vi "Host-Top-Level.vi"() -> ()   [LabVIEW 2015]
uses:
  <vilib>/rvi/interface/RandomDataEmulation/nirviRandomDataOpen.vi
  <vilib>/rvi/interface/common/niFpgaCacheSessionInfoDynamic.vi
  <vilib>/Utility/error.llb/Error Cluster From Error Code.vi
  <vilib>/rvi/errors/niLvFpgaAdjustHostInterfaceError.vi
  <vilib>/FPGAPlugInAG/Dynamic/niLvFpga_Close_Dynamic.vi
  <vilib>/rvi/interface/nirviOpenFPGA/nirviOpenFPGA.xnode
  FPGA-SRAM-Top-Level.vi
  <vilib>/rvi/interface/nirviMethod/nirviMethod.xnode
  <vilib>/rvi/interface/nirviCloseFPGA/nirviCloseFPGA.xnode
  <vilib>/FPGAPlugInAG/Dynamic/niLvFpga_WriteFifo_Dynamic.vi
  <vilib>/rvi/errors/niLvFpgaMergeErrorWithErrorCode.vi
  <vilib>/FPGAPlugInAG/Dynamic/niLvFpga_ReadFifo_Dynamic.vi
panel:
  out "error out":errorcluster
  in  "error in":errorcluster
  in  "# of \nElements":u32=2
  in  "Start\nAddress":u32
  out "Data Out":u64[](array[numeric])
  in  "Write Memory":bool
  in  "Data":u64[](array[numeric])=[10, 11, 12, 13, 14]
  in  "Exit":bool
  in  "Read Memory":bool
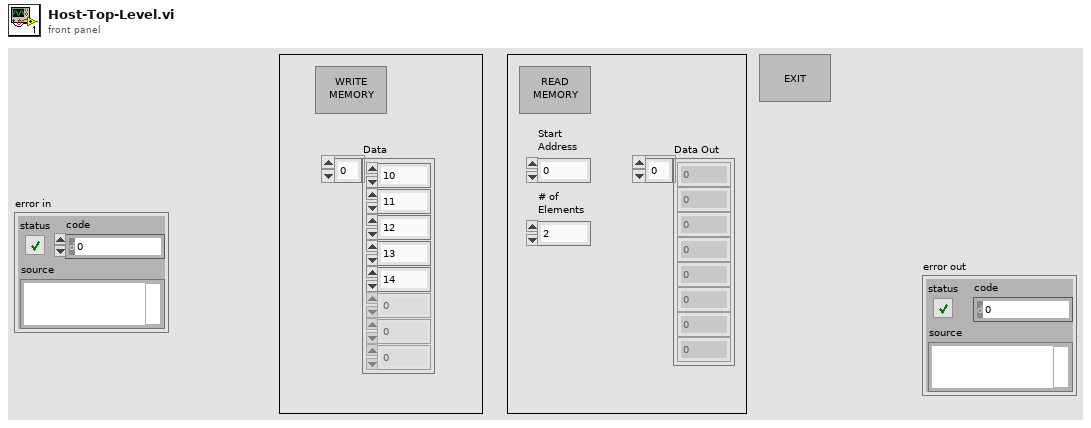
[diagram p1: front panel]
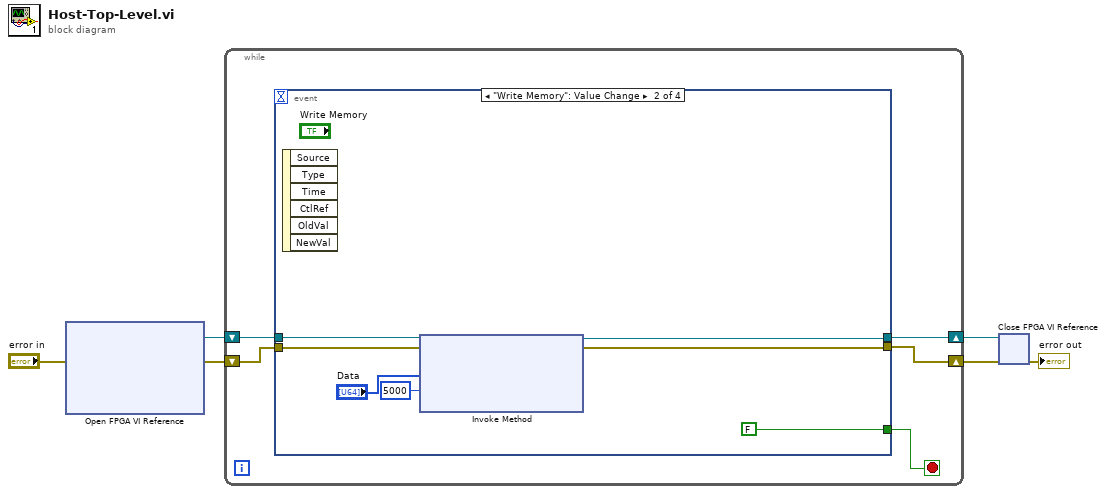
[diagram p0: block diagram]
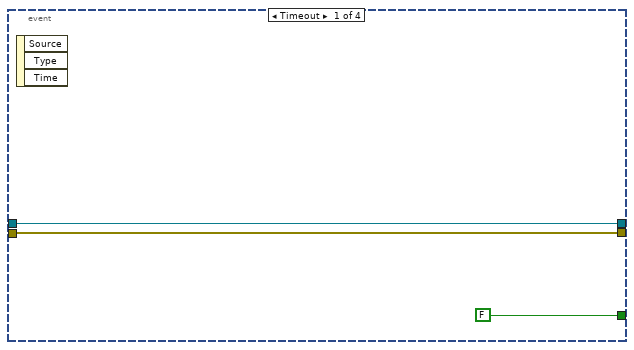
[diagram p2: hidden frame]
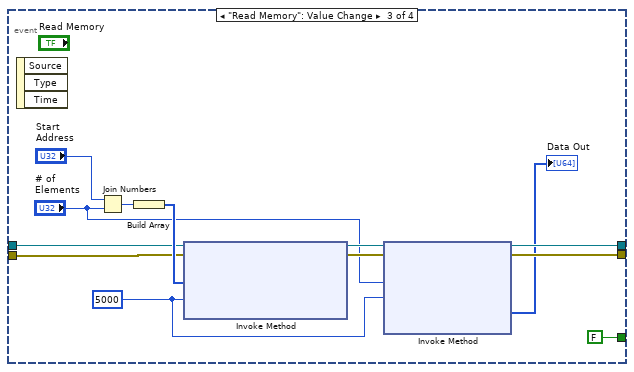
[diagram p3: hidden frame]
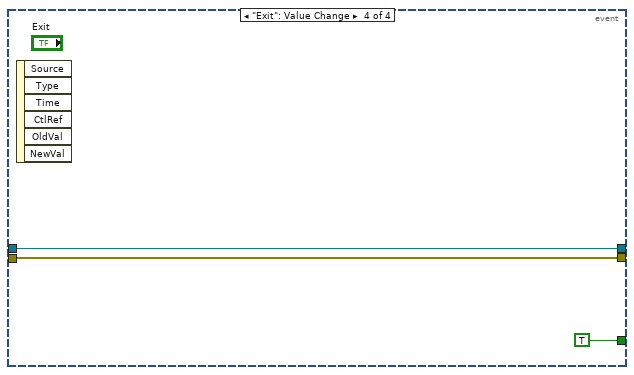
[diagram p4: hidden frame]
diagram:
  n1 = xnode "Open FPGA VI Reference"("error in"="error in") -> ("FPGA VI Reference Out"=w4:refnum<k20>, "error out"=w5:errorcluster)  [unwired: 1 in]
  n2 = while {
    shift-right: [w8] -> w1
    shift-left: w5 -> [w7]
    shift-right: [w9] -> w2
    shift-left: w4 -> [w10]
    stop <- w11 stop-if-true
    n3 = event shown="[1] \"Write Memory\": Value Change" {
      selector: _ -> [_ _ _ _]
      dyn-events: _ -> [_ _ _ _]
      timeout: _ -> [_ _ _ _]
      tunnel: [FALSE ("stop") FALSE ("stop") FALSE ("stop") TRUE ("stop")] -> w11
      tunnel: w10 -> [w13 w21 w31 w36]
      tunnel: [w13 w20 w26 w36] -> w9
      tunnel: [w12 w19 w25 w35] -> w8
      tunnel: w7 -> [w12 w18 w30 w35]
      event Timeout {
        n4 = event-data() -> ()  [unwired: 1 in, 3 out]
      }
      event "Write Memory": Value Change {
        n5 = event-data() -> ()  [unwired: 1 in, 6 out]
        n6 = xnode "Invoke Method"("FPGA VI Reference In"=w21, "error in"=w18, "Data"="Data", "Timeout (ms)"=5000) -> ("FPGA VI Reference Out"=w20:refnum<k20>, "error out"=w19:errorcluster)  [unwired: 1 out]
      }
      event "Read Memory": Value Change {
        w23 = 5000 ("Timeout (ms)")
        n7 = event-data() -> ()  [unwired: 1 in, 3 out]
        n8 = Join Numbers(hi="Start\nAddress", lo="# of \nElements") -> ((hi.lo)=w33:u64)
        n9 = Build Array(w33) -> (w32:u64[])
        n10 = xnode "Invoke Method"("FPGA VI Reference In"=w31, "error in"=w30, "Data"=w32, "Timeout (ms)"=w23) -> ("FPGA VI Reference Out"=w28:refnum<k20>, "error out"=w27:errorcluster)  [unwired: 1 out]
        n11 = xnode "Invoke Method"("FPGA VI Reference In"=w28, "error in"=w27, "Number of Elements"="# of \nElements", "Timeout (ms)"=w23) -> ("FPGA VI Reference Out"=w26:refnum<k20>, "error out"=w25:errorcluster, "Data"=→"Data Out":u64[])  [unwired: 1 out]
      }
      event "Exit": Value Change {
        n12 = event-data() -> ()  [unwired: 1 in, 6 out]
      }
    }
  }
  n13 = xnode "Close FPGA VI Reference"("FPGA VI Reference In"=w2, "error in"=w1) -> ("error out"=→"error out":errorcluster)
